vi "GET_info_METEO.vi"(7 "Update GHI":bool, 8 "error in":errorcluster, 9 "set Temp":dbl=100.0 format="%#_13g", 10 "set GHI":dbl=100.0 format="%#_13g", 11 "connection ID in":refnum<k5>) -> (0 "error out":errorcluster, 1 "read Temp":dbl, 2 "read GHI":dbl, 3 "connection ID out":refnum<k5>)   [LabVIEW 2021]
uses:
  Example TCP.lvlib
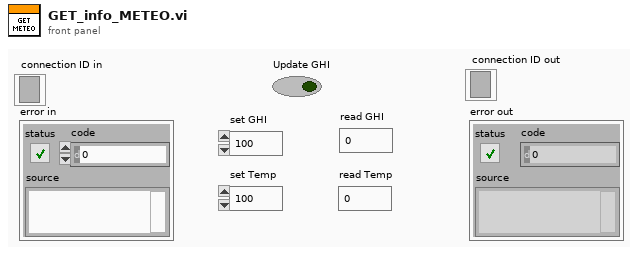
[diagram p1: front panel]
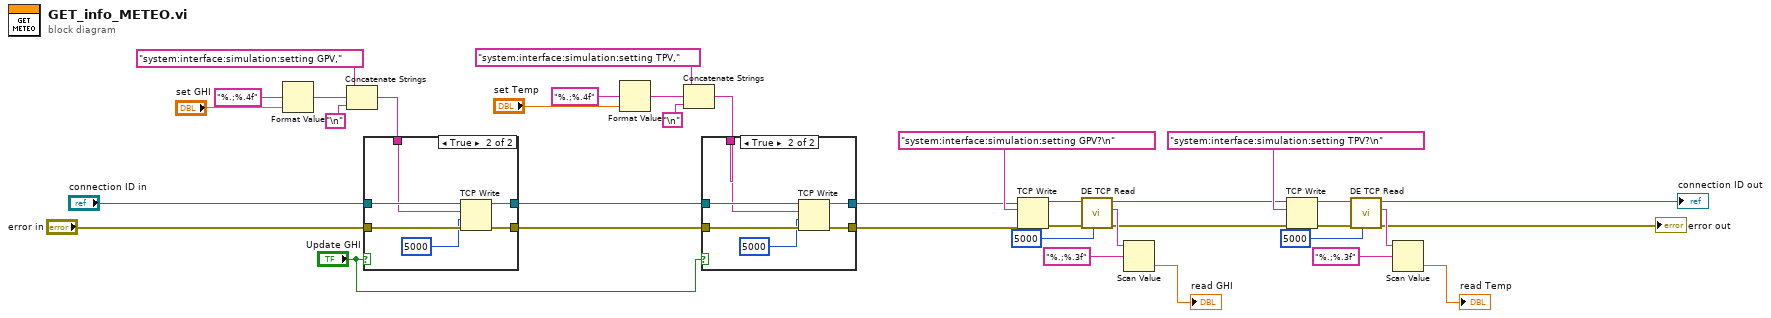
[diagram p0: block diagram]
diagram:
  n1 = Format Value(format string="%.;%.4f", value (0)="set GHI") -> (output string=w37:string)  [unwired: 1 in]
  n2 = Concatenate Strings("system:interface:simulation:setting GPV," ("data in"), w37, "\n" ("string")) -> (w28:string)
  n3 = case shown="True" "Update GHI" {
    tunnel: "error in" -> [w38 w45]
    tunnel: "connection ID in" -> [w39 w44]
    tunnel: w28 -> [_ w43]
    tunnel: [w39 w42] -> w21
    tunnel: [w38 w41] -> w20
    frame False {
    }
    frame True {
      n4 = TCP Write(connection ID=w44, data in=w43, error in (no error)=w45, 9:5000 ("timeout ms (25000)")) -> (connection ID out=w42:refnum<k5>, error out=w41:errorcluster)  [unwired: 1 out]
    }
  }
  n5 = Format Value(format string="%.;%.4f", value (0)="set Temp") -> (output string=w27:string)  [unwired: 1 in]
  n6 = Concatenate Strings("system:interface:simulation:setting TPV," ("data in"), w27, "\n" ("string")) -> (w23:string)
  n7 = case shown="True" "Update GHI" {
    tunnel: w20 -> [w46 w53]
    tunnel: w21 -> [w47 w52]
    tunnel: w23 -> [_ w51]
    tunnel: [w47 w50] -> w8
    tunnel: [w46 w49] -> w7
    frame False {
    }
    frame True {
      n8 = TCP Write(connection ID=w52, data in=w51, error in (no error)=w53, 9:5000 ("timeout ms (25000)")) -> (connection ID out=w50:refnum<k5>, error out=w49:errorcluster)  [unwired: 1 out]
    }
  }
  n9 = TCP Write(connection ID=w8, data in="system:interface:simulation:setting GPV?\n", error in (no error)=w7) -> (connection ID out=w33:refnum<k5>, error out=w32:errorcluster)  [unwired: 1 in, 1 out]
  n10 = call "DE TCP Read.vi"("timeout ms (25000)"=5000, "error in (no error)"=w32, "Connection ID in"=w33) -> ("error out"=w12:errorcluster, "TCP Read data"=w31:string, "Connection ID out"=w13:refnum<k5>)  [unwired: 6 in]
  n11 = Scan Value(string=w31, format string="%.;%.3f") -> (value=→"read GHI":dbl)  [unwired: 1 in, 1 out]
  n12 = TCP Write(connection ID=w13, data in="system:interface:simulation:setting TPV?\n", error in (no error)=w12) -> (connection ID out=w18:refnum<k5>, error out=w17:errorcluster)  [unwired: 1 in, 1 out]
  n13 = call "DE TCP Read.vi"("timeout ms (25000)"=5000, "error in (no error)"=w17, "Connection ID in"=w18) -> ("error out"=→"error out":errorcluster, "TCP Read data"=w16:string, "Connection ID out"=→"connection ID out":refnum<k5>)  [unwired: 6 in]
  n14 = Scan Value(string=w16, format string="%.;%.3f") -> (value=→"read Temp":dbl)  [unwired: 1 in, 1 out]
